vi "DSF.Engine.Pointer.Status.Builder.State.Read.0D.vi"(8 "error in (no error)":errorcluster, 11 "Builder State Pointer in":refnum<class "DSF.Engine.Pointer.Status.Builder.State.lvclass">) -> (0 "error out":errorcluster, 2 "state":T1, 3 "Builder State Pointer out":refnum<class "DSF.Engine.Pointer.Status.Builder.State.lvclass">)   [LabVIEW 2017, in "DSF.Engine.lvlib" / "DSF.Engine.Pointer.Status.Builder.State.lvclass"]
uses:
  Pointer/DSF.Engine.Pointer.Status.Builder.State.lvclass
  C:/Git/DSF/Built/Memory/Memory Manager.lvlibp/1abvi3w/vi.lib/National Instruments/Memory Manager/Classes/Pointer/Memory.Pointer.lvclass
  Interface/DSF.Engine.Interface.Builder.Command.ctl
  Built/Memory/Memory Manager.lvlibp/1abvi3w/vi.lib/National Instruments/Memory Manager/Classes/Pointer/Memory.Pointer.Read.0D.U8.vi
  Built/Memory/Memory Manager.lvlibp/1abvi3w/vi.lib/National Instruments/Memory Manager/Classes/Pointer/Memory.Pointer.lvclass
  Interface/DSF.Engine.Interface.Builder.lvclass
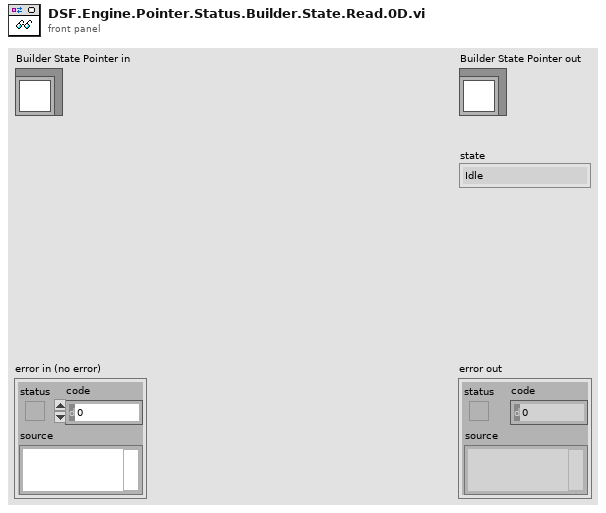
[diagram p1: front panel]
types:
  T1 = typedef "DSF.Engine.lvlib/DSF.Engine.Interface.Builder.lvclass/DSF.Engine.Interface.Builder.Command.ctl" = enum8{"Idle", "Initialize", "Build Buffer", "Parse Buffer", "Shutdown"}
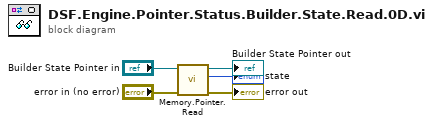
[diagram p0: block diagram]
diagram:
  n1 = call-poly "Memory.Pointer.Read.vi"("error in (no error)"="error in (no error)", "Pointer in"="Builder State Pointer in") -> ("error out"=→"error out":errorcluster, "value out"=→"state":u8, "Pointer out"=→"Builder State Pointer out":refnum<class "DSF.Engine.Pointer.Status.Builder.State.lvclass">)  [unwired: 6 in, 1 out]
